vi "Write Data.vi"(0 "UART Driver in":refnum<class "UART Driver.lvclass">, 1 "Port Number":u8, 5 "Tx Data":string, 11 "error in":errorcluster) -> (4 "UART Driver out":refnum<class "UART Driver.lvclass">, 15 "error out":errorcluster)   [LabVIEW 2012, in "UART_Host_Driver.lvlib" / "UART Driver.lvclass"]
doc: "Writes the data from the write buffer to the device or interface specified by the Channel Number.\n\nMust call UART Initialize.vi and UART Configure Port.vi prior to calling UART Write Data.vi.\n\nNote: Port Number 255 means to transmit to all of the ports configured in the UART Initialize.vi."
uses:
  UART Driver.lvclass
  Typedefs/FPGA VI Reference.ctl
  UART Driver.lvclass/UART Driver.ctl
  FPGA/UART/UART_Command.ctl
  <vilib>/Utility/error.llb/Error Cluster From Error Code.vi
  <vilib>/rvi/errors/niLvFpgaAdjustHostInterfaceError.vi
  <vilib>/rvi/interface/nirviMethod/nirviMethod.xnode
  UART_Host_Driver.lvlib
  FPGA/UART/UART_Firmware.lvlib
  <vilib>/FPGAPlugInAG/Dynamic/niLvFpga_WriteFifo_Dynamic.vi
  <vilib>/rvi/errors/niLvFpgaMergeErrorWithErrorCode.vi
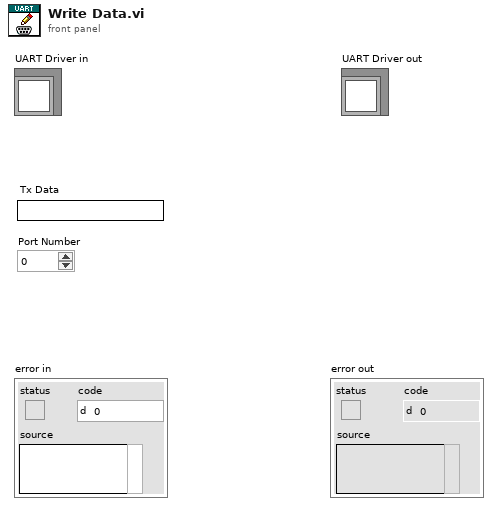
[diagram p1: front panel]
types:
  T1 = typedef "UART_Host_Driver.lvlib/FPGA VI Reference.ctl" = refnum<k20>
  T2 = typedef "UART_Firmware.lvlib/UART_Command.ctl" = enum8{"None", "Tx", "SetBaud_High", "SetBaud_Low", "SetCharLength", "SetParity", "SetStopBits", "SetSpacing_High", "SetSpacing_Low"}
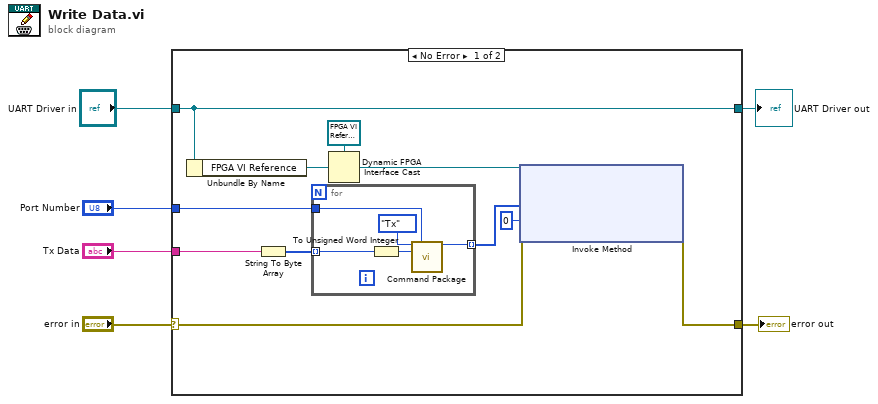
[diagram p0: block diagram]
diagram:
  n1 = case shown="No Error" "error in" {
    selector: "error in" -> [w13 w24]
    tunnel: [w10 w24] -> w5
    tunnel: [w17 w23] -> w3
    tunnel: "UART Driver in" -> [w17 w23]
    tunnel: "Tx Data" -> [w12 _]
    tunnel: "Port Number" -> [w9 _]
    frame No Error {
      n2 = Unbundle By Name(w17) -> ("FPGA VI Reference"=w16:refnum<k20>)
      n3 = String To Byte Array(string=w12) -> (unsigned byte array=w11:u8[])
      n4 = for {
        tunnel: w11 -> [w22] mode=indexing
        tunnel: [w20] -> w8 mode=indexing
        tunnel: w9 -> [w18]
        n5 = To Unsigned Word Integer(number=w22) -> (unsigned 16bit integer=w21:u16)
        n6 = call "Command Package.vi"("UART_Command"=UART_Command."Tx", "Channel Number"=w18, "Cmd_data"=w21) -> ("Cmd_package"=w20:u32)  [unwired: 12 in]
      }
      n7 = Dynamic FPGA Interface Cast(Session In=T1 refnum ("FPGA VI Reference"), Type=w16) -> (Session Out=w14:T1)
      n8 = xnode "Invoke Method"("FPGA VI Reference In"=w14, "error in"=w13, "Data"=w8, "Timeout (ms)"=0) -> ("error out"=w10:errorcluster)  [unwired: 2 out]
    }
    frame Error {
    }
  }
  "error out" <- w5
  "UART Driver out" <- w3
